vi "lookup_node_predecessors_by_id.vi"(8 "error in (no error)":errorcluster, 10 "node":refnum<class "ID.lvclass">, 11 "Graph in":refnum<class "DiGraph.lvclass">) -> (0 "error out":errorcluster, 2 "predecessors":set{refnum<class "ID.lvclass">}(c389))   [LabVIEW 2020, in "graph.lvlib" / "DiGraph.lvclass"]
uses:
  DiGraph.lvclass
  ID/ID.lvclass
  DiGraph.lvclass/DiGraph.ctl
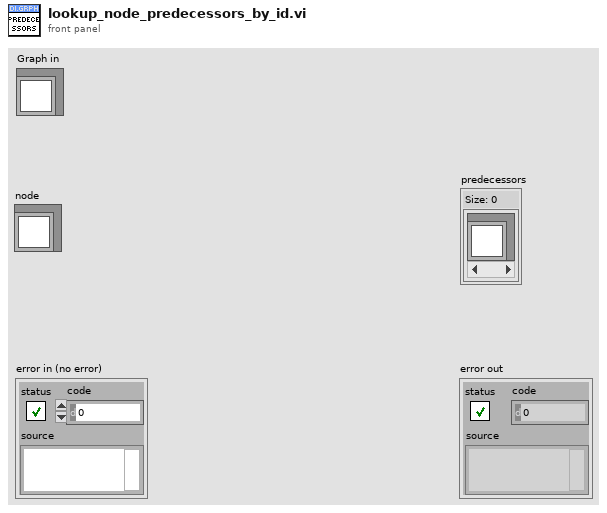
[diagram p1: front panel]
types:
  T1 = map{refnum<class "ID.lvclass">, set{refnum<class "ID.lvclass">}}
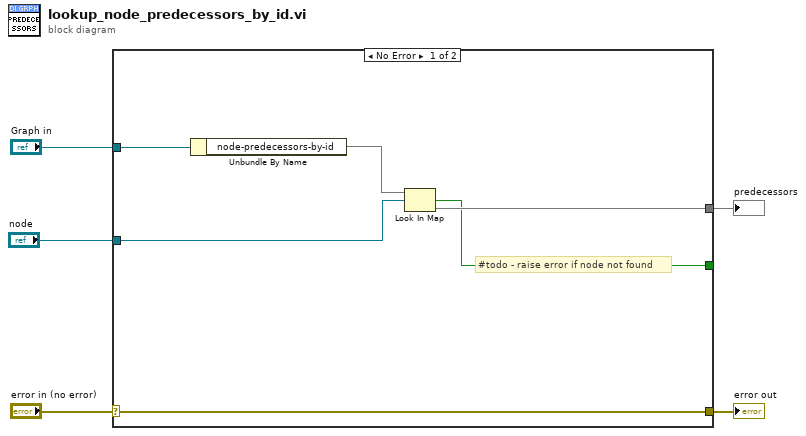
[diagram p0: block diagram]
diagram:
  n1 = case shown="No Error" "error in (no error)" {
    selector: "error in (no error)" -> [w11 w12]
    tunnel: [w11 w12] -> w4
    tunnel: "Graph in" -> [w10 _]
    tunnel: "node" -> [w9 _]
    tunnel: [w8 _] -> w1
    tunnel: [w6 _] -> _
    frame No Error {
      # "#todo - raise error if node not found"
      n2 = Unbundle By Name(w10) -> ("node-predecessors-by-id"=w7:T1)
      n3 = Look In Map(map=w7, key=w9) -> (key not found?=w6:bool, value=w8:set{refnum<class "ID.lvclass">})  [unwired: 1 in]
    }
    frame Error {
    }
  }
  "error out" <- w4
  "predecessors" <- w1
